vi "Timer.vi"() -> (2 "One second has passed":bool)   [LabVIEW 2015]
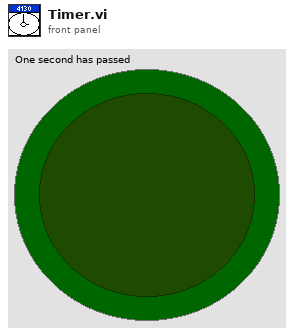
[diagram p1: front panel]
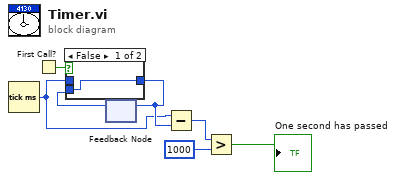
[diagram p0: block diagram]
diagram:
  n1 = Tick Count (ms)() -> (millisecond timer value=w3:u32)
  n2 = First Call?() -> (First Call?: T/F=w7:bool)
  n3 = feedback #1() -> (w6:u32)  [unwired: 1 in]
  n4 = case shown="False" w7 {
    tunnel: w3 -> [_ w9]
    tunnel: [w8 w9] -> w4
    tunnel: w6 -> [w8 _]
    frame False {
    }
    frame True {
    }
  }
  n5 = feedback-in #1(w4) -> ()
  n6 = Subtract(x=w3, y=w4) -> (x-y=w5:u32)
  n7 = Greater?(x=w5, y=u32 1000) -> (0:→"One second has passed":bool)
